vi "Motor Ramp.vi"(10 "Command limit":dbl, 11 "Joystick in":dbl) -> (3 "Joystick out":dbl)   [LabVIEW 2015]
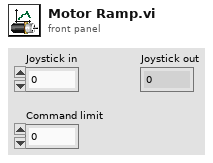
[diagram p1: front panel]
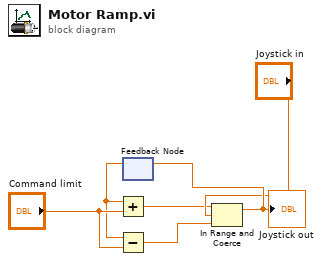
[diagram p0: block diagram]
diagram:
  n1 = feedback #1() -> (w4:dbl)  [unwired: 1 in]
  n2 = Add(x=w4, y="Command limit") -> (x+y=w2:dbl)
  n3 = Subtract(x=w4, y="Command limit") -> (x-y=w1:dbl)
  n4 = In Range and Coerce(upper limit=w2, x="Joystick in", lower limit=w1) -> (coerced(x)=w6:dbl)  [unwired: 1 out]
  "Joystick out" <- w6
  n5 = feedback-in #1(w6) -> ()
